vi "Practica 12 - Formula General.vi"() -> ()   [LabVIEW 2020]
panel:
  out "TIPO DE RAIZ":string
  out "RAIZ 2":dbl
  out "RAIZ 1":dbl
  in  "C":dbl
  in  "B":dbl
  in  "A":dbl
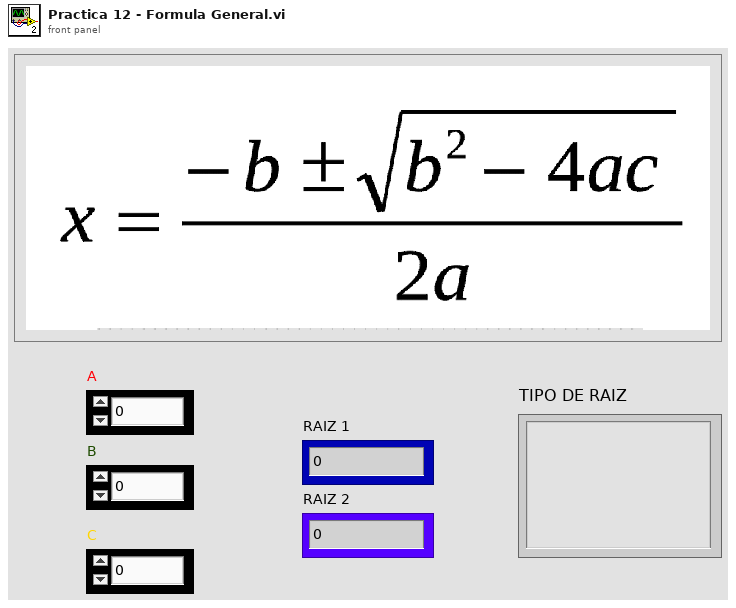
[diagram p1: front panel]
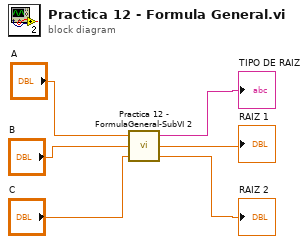
[diagram p0: block diagram]
diagram:
  n1 = call "Practica 12 - FormulaGeneral-SubVI 2.vi"("C"="C", "B"="B", "A"="A") -> ("RAIZ 2"=→"RAIZ 2":dbl, "RAIZ 1"=→"RAIZ 1":dbl, "TIPO DE RAIZ"=→"TIPO DE RAIZ":string)
